vi "nmap ping ip array.vi"(4 "error in (no error)":errorcluster, 7 "IP Addresses to search":string[](array[string])) -> (0 "error out":errorcluster, 1 "All on?":bool, 2 "IP Addresses on network":string[](array[string]), 3 "Computers not on":string[](array[string]))   [LabVIEW 2013]
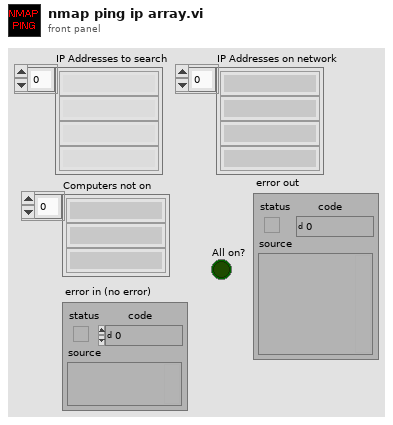
[diagram p1: front panel]
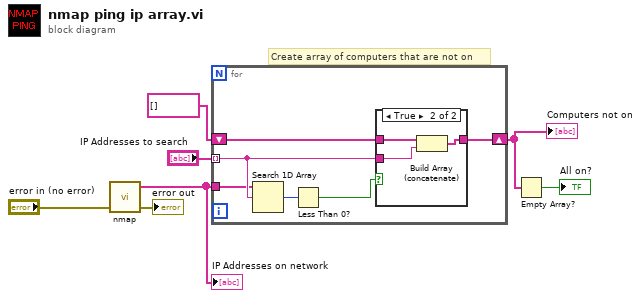
[diagram p0: block diagram]
diagram:
  # "Create array of computers that are not on"
  n1 = call "nmap.vi"("error in (no error)"="error in (no error)") -> ("error out"=→"error out":errorcluster, "IPs"=w3:string[])  [unwired: 3 in]
  "IP Addresses on network" <- w3
  n2 = for {
    tunnel: "IP Addresses to search" -> [w11] mode=indexing
    shift-right: [w12] -> w6
    shift-left: string[] [] -> [w13]
    tunnel: w3 -> [w10]
    n3 = Search 1D Array(1D array=w10, element=w11) -> (index of element=w9:i32)  [unwired: 1 in]
    n4 = Less Than 0?(x=w9) -> (x < 0?=w8:bool)
    n5 = case shown="True" w8 {
      tunnel: w13 -> [w14 w17]
      tunnel: w11 -> [_ w16]
      tunnel: [w14 w15] -> w12
      frame False {
      }
      frame True {
        n6 = Build Array (concatenate)(w17, w16) -> (w15:string[])
      }
    }
  }
  "Computers not on" <- w6
  n7 = Empty Array?(array=w6) -> (empty?=→"All on?":bool)
